vi "Manipulator PWM-y.vi"(7 "X axis":i32, 8 "output cluster":T1, 10 "Z axis":i32, 11 "Y axis":i32) -> (1 "wyj pwm manip.":T2)   [LabVIEW 2015]
uses:
  wyj manip.ctl
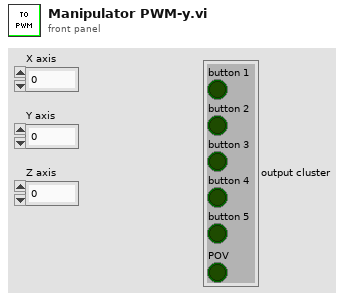
[diagram p1: front panel]
types:
  T1 = typedef "wyj manip.ctl" = cluster{"button 1":bool, "button 2":bool, "button 3":bool, "button 4":bool, "button 5":bool, "POV":bool}
  T2 = cluster{"pwm 1":i16, "pwm 2":i16, "pwm 3":i16, "pwm 4":i16, "pwm 5":i16, "pwm 6":i16, "pwm 7":i16}
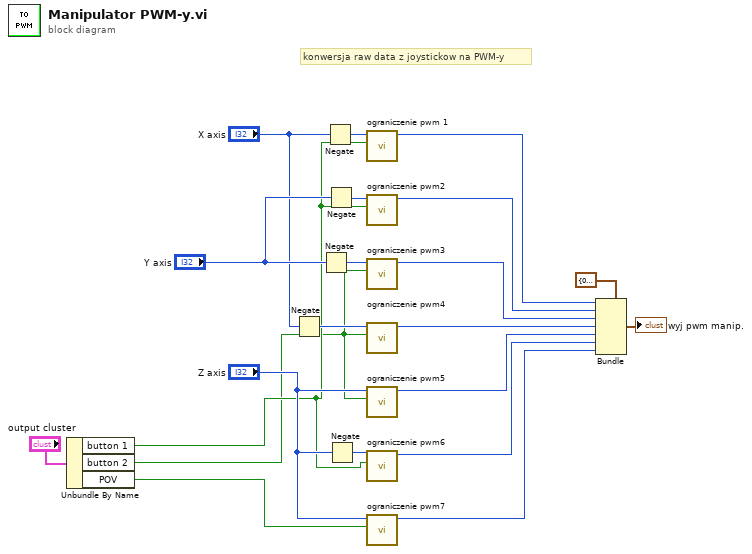
[diagram p0: block diagram]
diagram:
  # "konwersja raw data z joystickow na PWM-y"
  n1 = Unbundle By Name("output cluster") -> ("button 1"=w3:bool, "button 2"=w2:bool, "POV"=w1:bool)
  n2 = Negate(x="X axis") -> (-x=w15:i32)
  n3 = Negate(x="Y axis") -> (-x=w17:i32)
  n4 = Negate(x="X axis") -> (-x=w19:i32)
  n5 = Negate(x="Y axis") -> (-x=w18:i32)
  n6 = Negate(x="Z axis") -> (-x=w21:i32)
  n7 = call "ograniczenie pwm 1.vi"("button 1"=w3, "X axis"=w19) -> ("y"=w12:i16)  [unwired: 9 in]
  n8 = call "ograniczenie pwm2.vi"("button 1"=w3, "X axis"=w18) -> ("y"=w11:i16)  [unwired: 9 in]
  n9 = call "ograniczenie pwm3.vi"("button 1"=w2, "X axis"=w17) -> ("y"=w10:i16)  [unwired: 9 in]
  n10 = call "ograniczenie pwm4.vi"("button 1"=w2, "X axis"=w15) -> ("y"=w9:i16)  [unwired: 9 in]
  n11 = call "ograniczenie pwm5.vi"("button 1"=w2, "X axis"="Z axis") -> ("y"=w8:i16)  [unwired: 9 in]
  n12 = call "ograniczenie pwm6.vi"("button 1"=w3, "X axis"=w21) -> ("y"=w7:i16)  [unwired: 9 in]
  n13 = call "ograniczenie pwm7.vi"("button 1"=w1, "X axis"="Z axis") -> ("y"=w6:i16)  [unwired: 9 in]
  n14 = Bundle(cluster=T2 {"pwm 1"=0, "pwm 2"=0, "pwm 3"=0, "pwm 4"=0, "pwm 5"=0, "pwm 6"=0, "pwm 7"=0} ("output cluster"), "pwm 1"=w12, "pwm 2"=w11, "pwm 3"=w10, "pwm 4"=w9, "pwm 5"=w8, "pwm 6"=w7, "pwm 7"=w6) -> (→"wyj pwm manip.":T2)
